vi "Filtering - mirror mode.vi"(8 "error in (no error)":errorcluster) -> (0 "error out":errorcluster)   [LabVIEW 2026, in "Tests.lvlib"]
doc: "Integration test. Verifies that a single Log call fans out to every registered appender: registers three queue-mode relay appenders, logs one Info message, and asserts each appender's queue receives exactly one Statement with identical payload. Every gate except fan-out is held open (global threshold at floor, permissive filters, unbounded queues), so a missing element can only be a fan-out defect.\n\nImplements LMBR-T-030 -> SRS-019, SRS-028. Assert-level IDs: Test-ID-Assert-Checklist.md."
uses:
  Tests.lvlib
  src/TypeDefs/Severity.ctl
  <vilib>/addons/_JKI Toolkits/Caraya/classes/Assert/Assert Equal Value_Variant.vi
  <vilib>/addons/_JKI Toolkits/Caraya/classes/Assert/Assert True.vi
  <vilib>/addons/_JKI Toolkits/Caraya/classes/Test/Test.lvclass
  src/Lumberjack.lvlib
  src/Public/Logger.lvclass/Logger.lvclass
  <vilib>/addons/_JKI Toolkits/Caraya/classes/Assert/Assert.lvclass
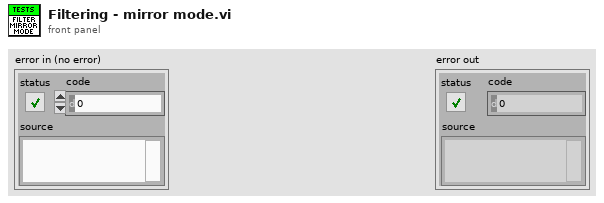
[diagram p1: front panel]
types:
  T1 = typedef "Lumberjack.lvlib/Severity.ctl" = enum16{"OFF", "FATAL", "ERROR", "WARN", "INFO", "DEBUG", "TRACE", "ALL"}
  T2 = typedef "Lumberjack.lvlib/Statement.ctl" = cluster{"timestamp":timestamp, "level":T1, "sourceTag":string, "originVI":string, "message":string}
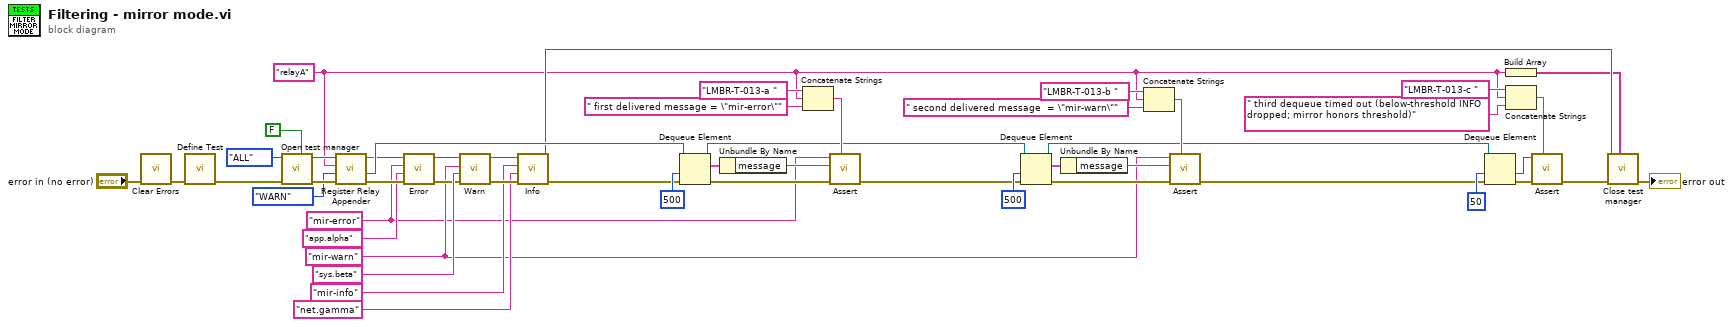
[diagram p0: block diagram]
diagram:
  w9 = "relayA"
  w7 = "mir-warn" ("message")
  w6 = "mir-error" ("message")
  n1 = call <vilib>:"Clear Errors.vi"("error in (no error)"="error in (no error)") -> ("error out"=w1:errorcluster)  [unwired: 5 in, 1 out]
  n2 = call <vilib>:"Define Test.vi"("error in (no error)"=w1) -> ("error out"=w51:errorcluster)  [unwired: 9 in, 1 out]
  n3 = call "Open test manager.vi"("enableDefaultFile"=FALSE, "error in (no error)"=w51, "globalThreshold"=Severity."ALL") -> ("error out"=w47:errorcluster, "Logger out"=w48:refnum<class "Logger.lvclass">)  [unwired: 7 in]
  n4 = call "Register Relay Appender.vi"("error in (no error)"=w47, "threshold"=Severity."WARN", "id in"=w9, "Logger in"=w48) -> ("error out"=w23:errorcluster, "relayQueue"=w26:refnum<queue>, "Logger out"=w15:refnum<class "Logger.lvclass">)  [unwired: 4 in, 1 out]
  n5 = call "Error.vi"("error in (no error)"=w23, "sourceTag"="app.alpha", "message"=w6, "Logger in"=w15) -> ("error out"=w20:errorcluster, "Logger out"=w14:refnum<class "Logger.lvclass">)  [unwired: 6 in]
  n6 = call "Warn.vi"("error in (no error)"=w20, "sourceTag"="sys.beta", "message"=w7, "Logger in"=w14) -> ("error out"=w19:errorcluster, "Logger out"=w17:refnum<class "Logger.lvclass">)  [unwired: 6 in]
  n7 = call "Info.vi"("error in (no error)"=w19, "sourceTag"="net.gamma", "message"="mir-info", "Logger in"=w17) -> ("error out"=w18:errorcluster, "Logger out"=w16:refnum<class "Logger.lvclass">)  [unwired: 6 in]
  n8 = Dequeue Element(queue=w26, timeout in ms (-1)=500, error in (no error)=w18) -> (queue out=w10:refnum<queue>, element=w32:T2, error out=w30:errorcluster)  [unwired: 1 out]
  n9 = Unbundle By Name(w32) -> ("message"=w31:string)
  n10 = Concatenate Strings("LMBR-T-013-a ", w9, " first delivered message = \"mir-error\"") -> (w27:string)
  n11 = call-poly <vilib>:"Assert.vi"("Label"=w27, "error in (no error)"=w30, "Actual"=w31, "Expected"=w6) -> ("error out"=w11:errorcluster)  [unwired: 6 in, 1 out]
  n12 = Dequeue Element(queue=w10, timeout in ms (-1)=500, error in (no error)=w11) -> (queue out=w4:refnum<queue>, element=w44:T2, error out=w39:errorcluster)  [unwired: 1 out]
  n13 = Unbundle By Name(w44) -> ("message"=w43:string)
  n14 = Concatenate Strings("LMBR-T-013-b ", w9, " second delivered message  = \"mir-warn\"") -> (w34:string)
  n15 = call-poly <vilib>:"Assert.vi"("Label"=w34, "error in (no error)"=w39, "Actual"=w43, "Expected"=w7) -> ("error out"=w5:errorcluster)  [unwired: 6 in, 1 out]
  n16 = Dequeue Element(queue=w4, timeout in ms (-1)=50, error in (no error)=w5) -> (timed out?=w40:bool, error out=w41:errorcluster)  [unwired: 2 out]
  n17 = Build Array(w9) -> (w8:string[])
  n18 = Concatenate Strings("LMBR-T-013-c ", w9, " third dequeue timed out (below-threshold INFO dropped; mirror honors threshold)") -> (w35:string)
  n19 = call-poly <vilib>:"Assert.vi"("Label"=w35, "error in (no error)"=w41, "True?"=w40) -> ("error out"=w46:errorcluster)  [unwired: 7 in, 1 out]
  n20 = call "Close test manager.vi"("queueIDList"=w8, "error in (no error)"=w46, "Logger in"=w16) -> ("error out"=→"error out":errorcluster)  [unwired: 6 in]
